vi "FactoryCreate.vi"(0 "reference in":refnum<class "ActorNode.lvclass">, 5 "error in (no error)":errorcluster) -> (14 "reference out":refnum<class "ActorNode.lvclass">, 19 "error out":errorcluster)   [LabVIEW 2016, in "ActorNode.lvclass"]
uses:
  <resource>/Framework/Providers/Open_GDS/UML/ActorNode_class/ActorNode.lvclass
  <resource>/Framework/Providers/Open_GDS/UML/ActorNode_class/ActorNode.lvclass/ActorNode.ctl
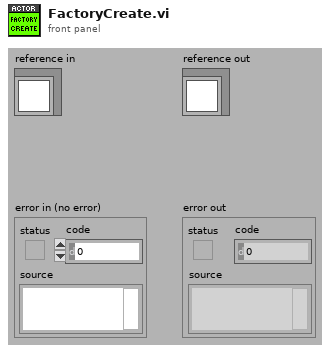
[diagram p1: front panel]
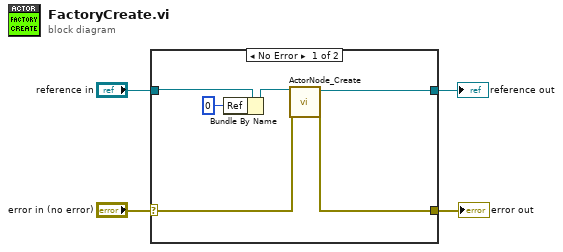
[diagram p0: block diagram]
diagram:
  n1 = case shown="No Error" "error in (no error)" {
    selector: "error in (no error)" -> [w9 w12]
    tunnel: [w8 w12] -> w3
    tunnel: [w7 w11] -> w1
    tunnel: "reference in" -> [w10 w11]
    frame No Error {
      n2 = Bundle By Name(cluster=w10, "Ref"=u32 0) -> (w6:refnum<class "ActorNode.lvclass">)
      n3 = call <resource>:"ActorNode_Create.vi"("reference"=w6, "error in (no error)"=w9) -> ("reference out"=w7:refnum<class "ActorNode.lvclass">, "error out"=w8:errorcluster)  [unwired: 16 in]
    }
    frame Error {
    }
  }
  "error out" <- w3
  "reference out" <- w1
